vi "High Speed Processing.vi"(8 "error in":errorcluster, 10 "Waveform Array":sgl[][](array[numeric]), 11 "DAQ Actor in":refnum<class "DAQ Actor.lvclass">) -> (0 "error out":errorcluster, 2 "Waveform Array":sgl[][](array[numeric]), 3 "DAQ Actor out":refnum<class "DAQ Actor.lvclass">)   [LabVIEW 2018, in "Data Acquisition.lvlib" / "DAQ Actor.lvclass"]
uses:
  DAQ Actor.lvclass
  DAQ Actor.lvclass/DAQ Actor.ctl
  TCP Server/TCP Writer Messages/Write Data to Stream Msg/Write Data to Conn Msg.lvclass/Write Data to Conn Msg.ctl
  <vilib>/ActorFramework/Message Enqueuer/Message Enqueuer.lvclass/Message Enqueuer.ctl
  <vilib>/ActorFramework/Message Enqueuer/Enqueue.vi
  TCP Server/TCP Writer Messages/Write Data to Stream Msg/Write Data to Conn Msg.lvclass
  C:/Program Files (x86)/National Instruments/LabVIEW 2018/vi.lib/ActorFramework/Message/Message.lvclass
  <vilib>/ActorFramework/Message Priority Queue/Priority Enqueue.vi
  Class DAQ Task/DAQ Task.lvclass
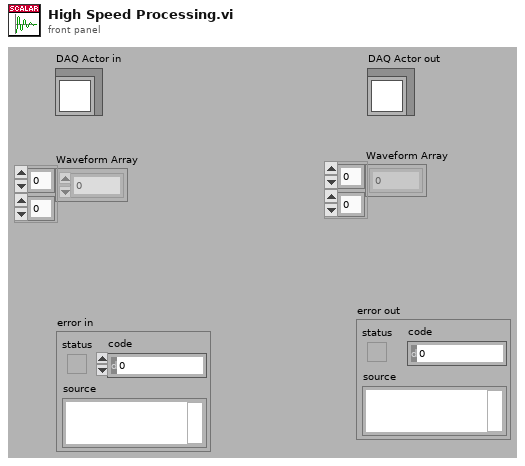
[diagram p1: front panel]
types:
  T1 = typedef "TE_Designator.ctl" = enum16{"High Speed", "Low Speed"}
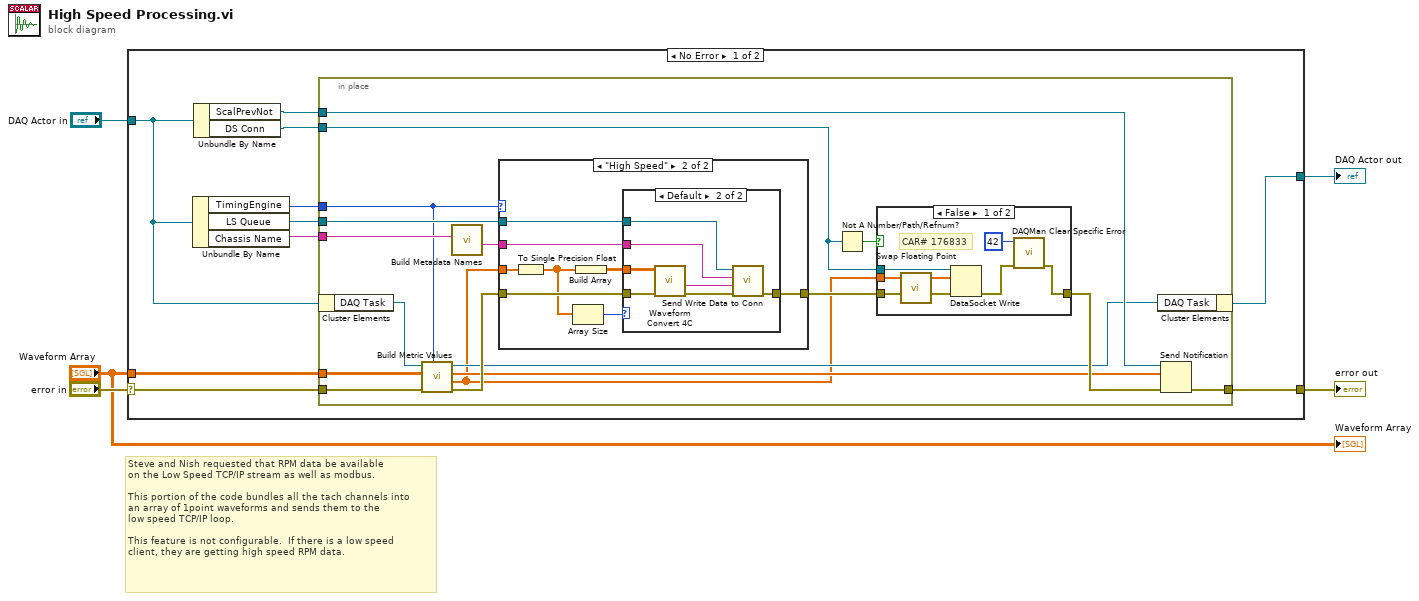
[diagram p0: block diagram]
diagram:
  # "Steve and Nish requested that RPM data be available\non the Low Speed TCP/IP stream as well as modbus.\n\nThis portion of the code bundles all the tach channels into\nan array of 1point waveforms and sends them to the\nlow speed TCP/IP loop.\n\nThis feature is not configurable.  If there is a low speed\nclient, they are getting high speed RPM data."
  n1 = case shown="No Error" "error in" {
    selector: "error in" -> [w10 w59]
    tunnel: [w15 w59] -> w5
    tunnel: [w8 w58] -> w4
    tunnel: "DAQ Actor in" -> [w9 w58]
    tunnel: "Waveform Array" -> [w12 _]
    frame No Error {
      n2 = Unbundle By Name(w9) -> ("TimingEngine"=w6:T1, "LS Queue"=w7:refnum<class "Message Enqueuer.lvclass">, "Chassis Name"=w11:string)
      n3 = Unbundle By Name(w9) -> ("ScalPrevNot"=w14:refnum<notifier>, "DS Conn"=w13:refnum<k13>)
      n4 = in-place {
        in-place-border: [w30] -> w15
        in-place-border: w14 -> [w29]
        in-place-border: w13 -> [w28]
        in-place-border: w12 -> [w27]
        in-place-border: w11 -> [w20]
        in-place-border: w10 -> [w23]
        in-place-border: w7 -> [w18]
        in-place-border: w6 -> [w17]
        n5 = in-place-cluster #1(w9) -> ("DAQ Task"=w22:refnum<class "DAQ Task.lvclass">)
        n6 = call "Build Metric Values.vi"("TimingEngine"=w17, "error in (no error)"=w23, "Waveform Array"=w27, "DAQ Task"=w22) -> ("error out"=w26:errorcluster, "Modbus Values"=w16:dbl[], "Ch Metrics"=w24:dbl[], "DAQ Task"=w21:refnum<class "DAQ Task.lvclass">)  [unwired: 4 in]
        n7 = call "Build Metadata Names.vi"("Chassis Name"=w20) -> ("Modbus Wfm"=w19:string)  [unwired: 6 in, 4 out]
        n8 = case shown="\"High Speed\"" w17 {
          tunnel: w26 -> [w33 w41]
          tunnel: [w33 w39] -> w25
          tunnel: w19 -> [_ w38]
          tunnel: w18 -> [_ w37]
          tunnel: w16 -> [_ w35]
          frame "Low Speed" {
          }
          frame "High Speed" {
            n9 = To Single Precision Float(number=w35) -> (single precision float=w34:sgl[])
            n10 = Array Size(array=w34) -> (size(s)=w40:i32)
            n11 = Build Array(w34) -> (w36:sgl[][])
            n12 = case shown="Default" w40 {
              tunnel: w41 -> [w42 w49]
              tunnel: [w42 w47] -> w39
              tunnel: w38 -> [_ w45]
              tunnel: w37 -> [_ w44]
              tunnel: w36 -> [_ w43]
              frame 0 {
              }
              frame Default {
                n13 = call "Waveform Convert 4C.vi"("error in"=w49, "Waveform Array"=w43) -> ("error out"=w48:errorcluster, "ModWfms"=w46:string)  [unwired: 8 in]
                n14 = call "Send Write Data to Conn.vi"("error in (no error)"=w48, "Data"=w46, "MetaData"=w45, "Message Enqueuer"=w44) -> ("error out"=w47:errorcluster)  [unwired: 6 in, 1 out]
              }
            }
          }
        }
        n15 = Not A Number/Path/Refnum?(number/path/refnum=w28) -> (NaN/Path/Refnum?=w32:bool)
        n16 = case shown="False" w32 {
          tunnel: w16 -> [w51 _]
          tunnel: w28 -> [w56 _]
          tunnel: w25 -> [w55 w57]
          tunnel: [w53 w57] -> w31
          frame False {
            # "CAR# 176833"
            n17 = call "Swap Floating Point.vi"("DBL Data"=w51) -> ("Swapped SGL Data"=w50:sgl[])  [unwired: 4 in]
            n18 = DataSocket Write(8:w55, 10:w50, 11:w56) -> (0:w54:errorcluster)  [unwired: 1 in, 2 out]
            n19 = call "DAQMan Clear Specific Error.vi"("error in"=w54, "code"=42) -> ("error out"=w53:errorcluster)  [unwired: 9 in]
          }
          frame True {
          }
        }
        n20 = in-place-cluster #1("DAQ Task"=w21) -> (w8:refnum<class "DAQ Actor.lvclass">)
        n21 = Send Notification(notification=w24, notifier=w29, error in (no error)=w31) -> (error out=w30:errorcluster)  [unwired: 1 out]
      }
    }
    frame Error {
    }
  }
  "error out" <- w5
  "DAQ Actor out" <- w4
  "Waveform Array" <- "Waveform Array"
